vi "CMD_Wait.vi"(1 "Line":string) -> (0 "Done":bool)   [LabVIEW 2017, in "Apple script.lvlib"]
uses:
  Apple script.lvlib
panel:
  in  "Parameters":i32[](array[numeric])=[1, 1]
  in  "Subcommands":string[](array[string])=["for", "until"]
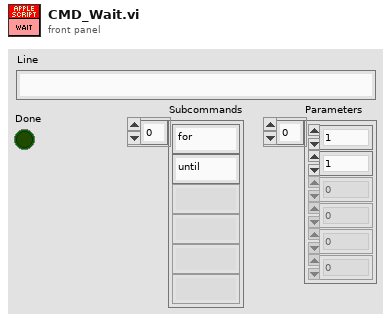
[diagram p1: front panel]
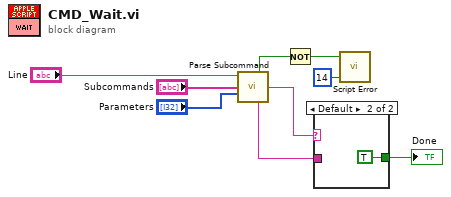
[diagram p0: block diagram]
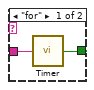
[diagram p2: hidden frame]
diagram:
  n1 = call "Parse Subcommand.vi"("Text In"="Line", "Subcommands"="Subcommands", "Parameters"="Parameters") -> ("Done"=w3:bool, "Subcommand"=w5:string, "Parameter 1"=w4:string)  [unwired: 6 in, 4 out]
  n2 = Not(x=w3) -> (.not. x?=w2:bool)
  n3 = case shown="Default" w5 {
    tunnel: w4 -> [w10 _]
    tunnel: [w11 TRUE ("Value")] -> w8
    frame "for" {
      n4 = call "Timer.vi"("Seconds (string)"=w10) -> ("Done"=w11:bool)
    }
    frame Default {
    }
  }
  "Done" <- w8
  n5 = call "Script Error.vi"("Error?"=w2, "Error Code"=14) -> ()  [unwired: 3 in, 1 out]
